vi "Default Settings.vi"(8 "error in (no error)":errorcluster, 11 "C4 Dispense in 2":refnum<class "8 Inch Iterative Dispense.lvclass">) -> (0 "error out":errorcluster, 3 "C4 Dispense out 2":refnum<class "8 Inch Iterative Dispense.lvclass">)   [LabVIEW 2016, in "8 Inch Iterative Dispense.lvclass"]
uses:
  8 Inch Iterative Dispense.lvclass
  D:/LabVIEW/20220413/UCSB-Gantry/V5/Classes/Routine/Dispense/Iterative Dispense/Iterative Dispense.lvclass
  D:/LabVIEW/20220413/UCSB-Gantry/V5/Classes/Routine/Dispense/Dispense.lvclass
  Iterative Dispense.lvclass/Iterative Dispense.ctl
  Read Speed.vi
  Read Number of Lines.vi
  Read Distance From Edges.vi
  Iterative Dispense.lvclass
  Dispense.lvclass
panel:
  # "This Routine does not Accept Settings"
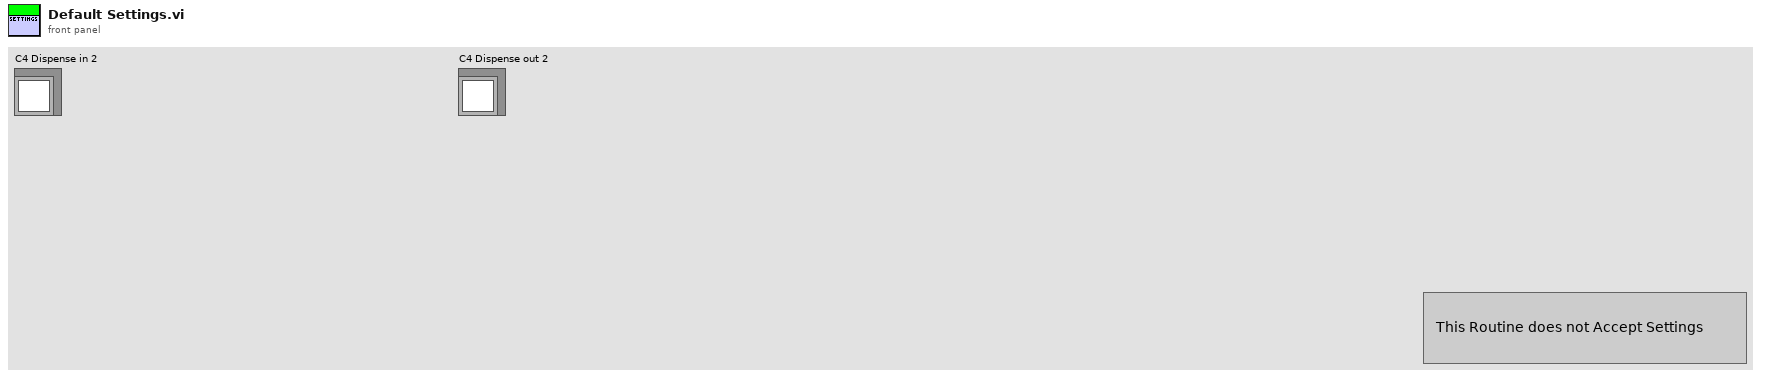
[diagram p1: front panel]
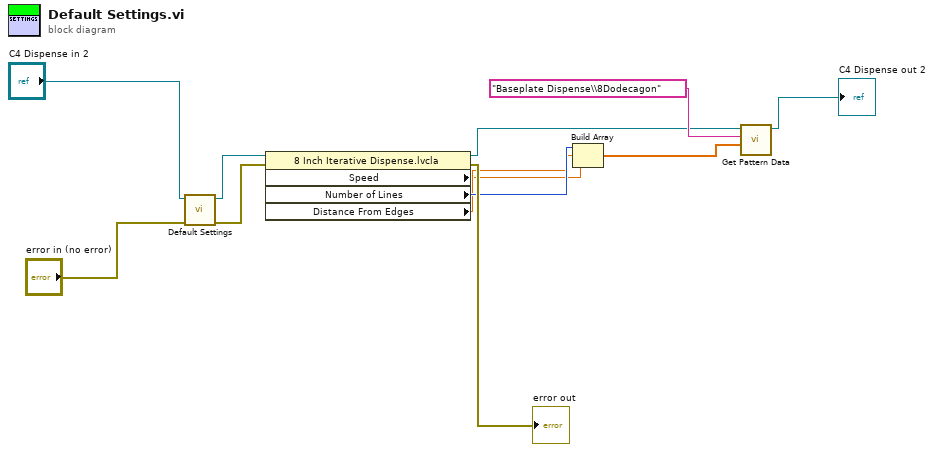
[diagram p0: block diagram]
diagram:
  n1 = call-parent "Default Settings.vi"("error in (no error)"="error in (no error)", "C4 Dispense in 2"="C4 Dispense in 2") -> ("error out"=w9:errorcluster, "C4 Dispense out 2"=w10:refnum<class "8 Inch Iterative Dispense.lvclass">)  [unwired: 8 in]
  n2 = property class="8 Inch Iterative Dispense.lvcla"(reference=w10, error in=w9) -> (reference out=w5:refnum<class "8 Inch Iterative Dispense.lvclass">, error out=→"error out":errorcluster, "Speed"=w1:dbl, "Number of Lines"=w3:i32, "Distance From Edges"=w2:dbl)
  n3 = Build Array(w3, w2, w1) -> (w7:dbl[])
  n4 = call "Get Pattern Data.vi"("File Name"=w7, "Folder Name"="Baseplate Dispense\\8Dodecagon", "Dispense.lvclass"=w5) -> ("Dispense Out"=→"C4 Dispense out 2":refnum<class "8 Inch Iterative Dispense.lvclass">)  [unwired: 8 in]
